vi "RC_Client 1.vi"(8 "error in (no error)":errorcluster, 11 "RC Type":T1) -> (0 "error out":errorcluster)   [LabVIEW 2019, in "RemoteControl.lvclass"]
uses:
  RemoteControl.lvclass
  Typedefs/RC Com Type--enum.ctl
  f0cea44e-82f5-4e56-b32e-d2cb384a2566.vi
  db51367f-c7f3-480a-b132-7f33093295d6.vi
  d8d5aeaf-e1b8-48f3-8146-827dda1e4654.vi
  f0cea44e-82f5-4e56-b32e-d2cb384a2566.vi/45cdd34d-a2c2-45d4-aff0-ceb647337bc5.vi
  db51367f-c7f3-480a-b132-7f33093295d6.vi/69d7a8c7-de6d-42ae-966a-0c233d979ea4.vi
  d8d5aeaf-e1b8-48f3-8146-827dda1e4654.vi/c7d4e3fa-5896-452d-a6ae-55c6b3b6fca4.vi
  <vilib>/Utility/LVClass/Get LV Class Name.vi
  <vilib>/JDP Science/JSONtext/JSON text to Variant.vi
  <userlib>/_OpenG.lib/numeric/numeric.llb/Random Number Within Range - I32__ogtk.vi
  <userlib>/_OpenG.lib/error/error.llb/Filter Error Codes (Array)__ogtk.vi
  <vilib>/JDP Science/JSONtext/LVClass Serializer/JSONtext LVClass Serializer.lvclass
panel:
  in  "milliseconds to wait":u32
  out "time (1 message) (s)":dbl
  out "startup time (s)":dbl
  out "messages/s":dbl
  in  "remote port":u16=6341
  in  "address":string
  out "Response":string
  out "Messages":i32
  in  "Stop":bool
  out "Command reponse":string
  out "Command":string
  out "meta data\n(available commands)":string
  # "CLIENT (API)"
  # "Connection info"
  # "Message Sent"
  # "Message Received"
  # "Metrics"
  # "1"
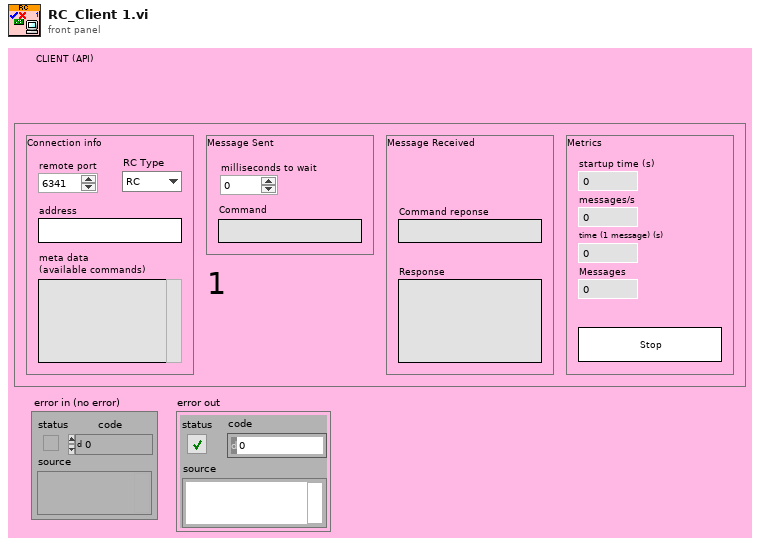
[diagram p1: front panel]
types:
  T1 = typedef "RemoteControl.lvclass/RC Com Type--enum.ctl" = enum16{"RC", "STM", "ZMQ"}
  T2 = cluster{"Command out":string, "Data out":variant, string}
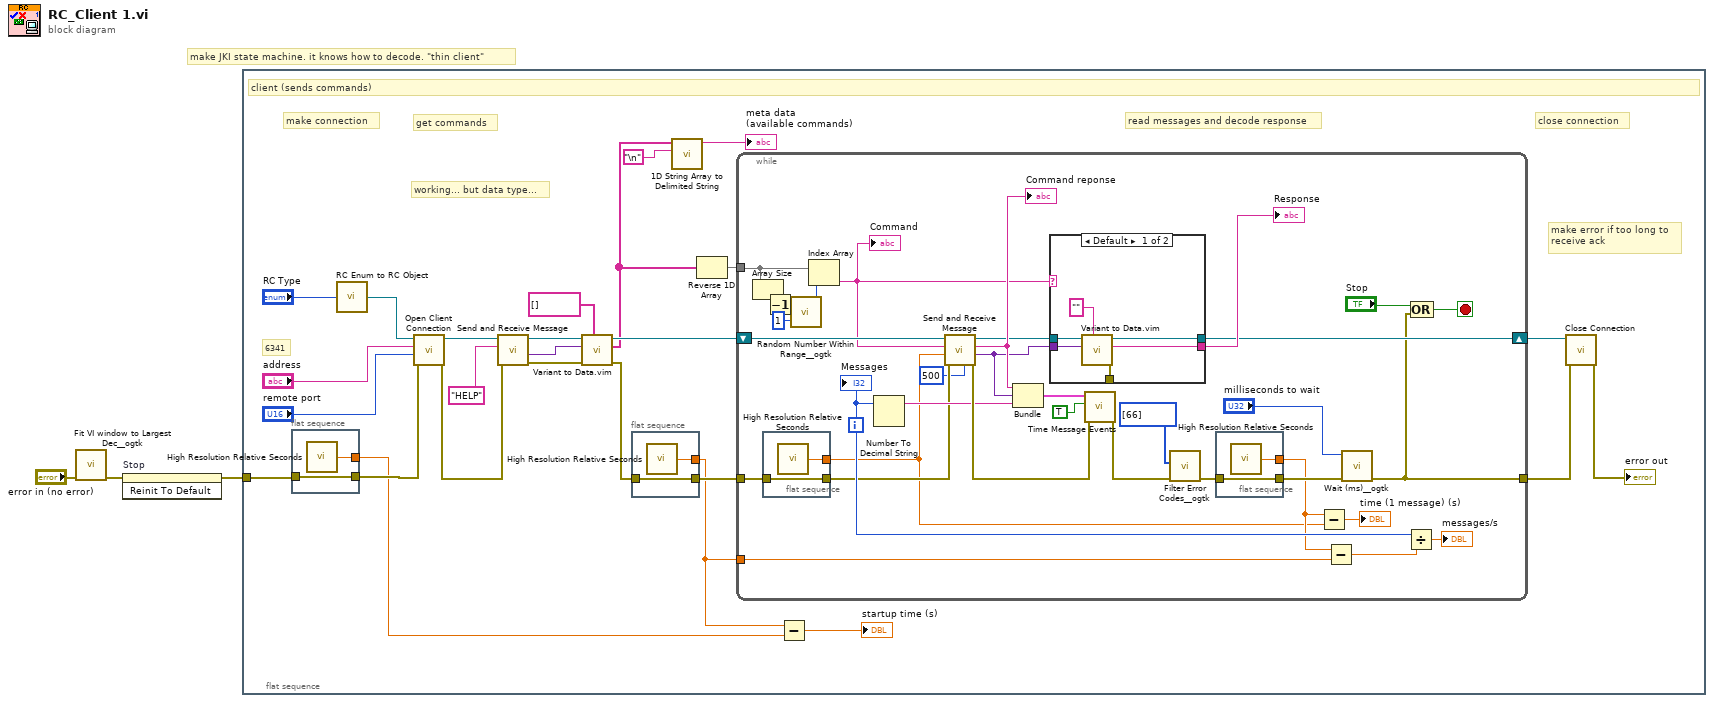
[diagram p0: block diagram]
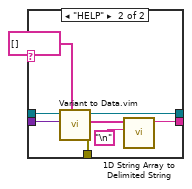
[diagram p2: hidden frame]
diagram:
  # "make JKI state machine. it knows how to decode. \"thin client\""
  n1 = call <userlib>:"Fit VI window to Largest Dec__ogtk.vi"("error in (no error)"="error in (no error)") -> ("error out"=w3:errorcluster)  [unwired: 5 in, 1 out]
  n2 = invoke on="Stop" class="Bool" method="Reinit To Default"(error in=w3) -> (error out=w2:errorcluster)  [unwired: 2 in, 2 out]
  n3 = flat-sequence {
    tunnel: w2 -> [w6]
    frame #0 {
      # "working... but data type..."
      # "close connection"
      # "read messages and decode response"
      # "get commands"
      # "make connection"
      # "6341"
      # "make error if too long to\nreceive ack"
      # "client (sends commands)"
      n4 = flat-sequence {
        tunnel: [w30] -> w5
        tunnel: [w31] -> w4
        tunnel: w6 -> [w30]
        frame #0 {
          n5 = call <vilib>:"High Resolution Relative Seconds.vi"() -> ("relative seconds"=w31:dbl)
        }
      }
      n6 = call "RC Enum to RC Object.vi"("RC Type"="RC Type") -> ("RemoteControl out"=w15:refnum<class "RemoteControl.lvclass">)
      n7 = call-dynamic "Open Client Connection.vi"("error in (no error)"=w5, "Port"="remote port", "address"="address", "RemoteControl in"=w15) -> ("error out"=w19:errorcluster, "RemoteControl out"=w17:refnum<class "RemoteControl.lvclass">)  [unwired: 6 in]
      n8 = call-dynamic "Send and Receive Message.vi"("error in (no error)"=w19, "Command"="HELP", "RemoteControl in"=w17) -> ("error out"=w16:errorcluster, "Data out"=w10:variant, "RemoteControl out"=w13:refnum<class "RemoteControl.lvclass">)  [unwired: 5 in, 1 out]
      n9 = call "Variant to Data.vim"("Data Type"=string[] [], "error in (no error)"=w16, "Data in"=w10, "RemoteControl in"=w13) -> ("error out"=w7:errorcluster, "Data out"=w8:string[], "RemoteControl out"=w12:refnum<class "RemoteControl.lvclass">)  [unwired: 5 in]
      n10 = flat-sequence {
        tunnel: [w32] -> w24
        tunnel: [w33] -> w20
        tunnel: w7 -> [w32]
        frame #0 {
          n11 = call <vilib>:"High Resolution Relative Seconds.vi"() -> ("relative seconds"=w33:dbl)
        }
      }
      n12 = call <vilib>:"1D String Array to Delimited String.vi"("delimiter"="\n", "string array"=w8) -> ("delimited string"=→"meta data\n(available commands)":string)  [unwired: 9 in]
      n13 = Reverse 1D Array(array=w8) -> (reversed array=w25:string[])
      n14 = while {
        tunnel: [w44] -> w29
        tunnel: w24 -> [w37]
        tunnel: w25 -> [w57]
        tunnel: w20 -> [w52]
        shift-right: [w47] -> w28
        shift-left: w12 -> [w66]
        i -> [w43]
        stop <- w42 stop-if-true
        n15 = Array Size(array=w57) -> (size(s)=w58:i32)
        n16 = flat-sequence {
          tunnel: [w68] -> w36
          tunnel: [w69] -> w35
          tunnel: w37 -> [w68]
          frame #0 {
            n17 = call <vilib>:"High Resolution Relative Seconds.vi"() -> ("relative seconds"=w69:dbl)
          }
        }
        n18 = Decrement(x=w58) -> (x-1=w56:i32)
        n19 = call-poly <userlib>:"Random Number Within Range__ogtk.vi"("High"=w56, "Low"=1) -> ("Random Number"=w60:i32)  [unwired: 3 in]
        n20 = Index Array(array=w57, index=w60) -> (element=w45:string)
        "Command" <- w45
        n21 = Number To Decimal String(number=w43) -> (decimal integer string=w46:string)  [unwired: 1 in]
        n22 = call-dynamic "Send and Receive Message.vi"("timeout (ms) [100]"=500, "error in (no error)"=w36, "Data"=w35, "Command"=w45, "RemoteControl in"=w66) -> ("error out"=w55:errorcluster, "Data out"=w48:variant, "Command out"=w64:string, "RemoteControl out"=w49:refnum<class "RemoteControl.lvclass">)  [unwired: 3 in]
        "Command reponse" <- w64
        n23 = Bundle("Command out"=w64, "Data out"=w48, w46) -> (w63:T2)  [unwired: 1 in]
        n24 = case shown="Default" w45 {
          tunnel: [w76 w80] -> w50
          tunnel: w49 -> [w75 w84]
          tunnel: w48 -> [w74 w83]
          tunnel: [w73 w82] -> w47
          tunnel: [w72 w78] -> _
          frame Default {
            n25 = call "Variant to Data.vim"("Data Type"="", "Data in"=w74, "RemoteControl in"=w75) -> ("error out"=w72:errorcluster, "Data out"=w76:string, "RemoteControl out"=w73:refnum<class "RemoteControl.lvclass">)  [unwired: 6 in]
          }
          frame "HELP" {
            n26 = call "Variant to Data.vim"("Data Type"=string[] [], "Data in"=w83, "RemoteControl in"=w84) -> ("error out"=w78:errorcluster, "Data out"=w81:string[], "RemoteControl out"=w82:refnum<class "RemoteControl.lvclass">)  [unwired: 6 in]
            n27 = call <vilib>:"1D String Array to Delimited String.vi"("delimiter"="\n", "string array"=w81) -> ("delimited string"=w80:string)  [unwired: 9 in]
          }
        }
        "Response" <- w50
        n28 = call "Time Message Events.vi"("error in (no error)"=w55, "Debug Mode"=TRUE, "Message in"=w63) -> ("error out"=w51:errorcluster)  [unwired: 6 in, 2 out]
        n29 = call-poly <userlib>:"Filter Error Codes__ogtk.vi"("Error In"=w51, "Error Codes to Filter"=i32[] [66]) -> ("Error Out"=w41:errorcluster)  [unwired: 7 in, 2 out]
        n30 = flat-sequence {
          tunnel: [w70] -> w40
          tunnel: [w71] -> w39
          tunnel: w41 -> [w70]
          frame #0 {
            n31 = call <vilib>:"High Resolution Relative Seconds.vi"() -> ("relative seconds"=w71:dbl)
          }
        }
        n32 = Subtract(x=w39, y=w35) -> (x-y=→"time (1 message) (s)":dbl)
        n33 = Subtract(x=w39, y=w52) -> (x-y=w38:dbl)
        n34 = call <userlib>:"Wait (ms)__ogtk.vi"("error in (no error)"=w40, "milliseconds to wait"="milliseconds to wait") -> ("error out"=w44:errorcluster)  [unwired: 8 in, 1 out]
        n35 = Divide(x=w43, y=w38) -> (x/y=→"messages/s":dbl)
        n36 = Compound Arithmetic op=OR("Stop", w44) -> (w42:bool)
        "Messages" <- w43
      }
      n37 = Subtract(x=w20, y=w4) -> (x-y=→"startup time (s)":dbl)
      n38 = call-dynamic "Close Connection.vi"("error in (no error)"=w29, "RemoteControl in"=w28) -> ("error out"=→"error out":errorcluster)  [unwired: 8 in, 1 out]
    }
  }
